vi "Read Active Cell Cell Justification.vi"(8 "error in (no error)":errorcluster, 11 "TreeControl.lvclass in":refnum<class "TreeControl.lvclass">) -> (0 "error out":errorcluster, 2 "CellJustify":enum16{"Left", "Center", "Right"}(ring), 3 "TreeControl.lvclass out":refnum<class "TreeControl.lvclass">)   [LabVIEW 2015, in "TreeControl.lvclass"]
uses:
  TreeControl.lvclass
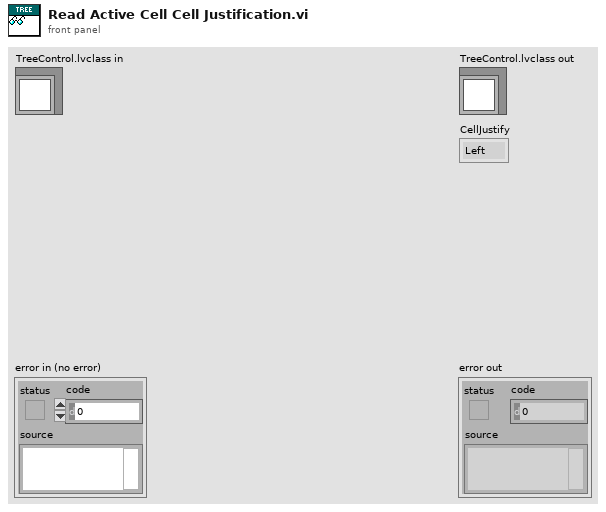
[diagram p1: front panel]
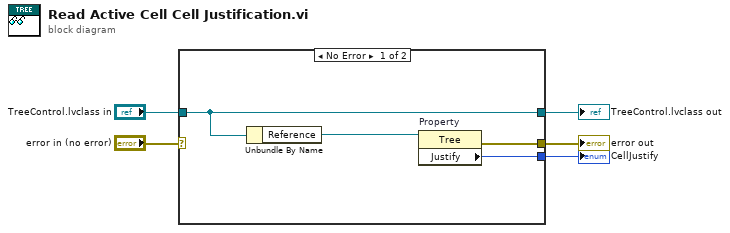
[diagram p0: block diagram]
diagram:
  n1 = case shown="No Error" "error in (no error)" {
    selector: "error in (no error)" -> [_ w11]
    tunnel: [w8 w11] -> w4
    tunnel: [w7 w10] -> w2
    tunnel: "TreeControl.lvclass in" -> [w7 w10]
    tunnel: [w9 _] -> w1
    frame No Error {
      n2 = Unbundle By Name(w7) -> ("Reference"=w6:refnum<vi>)
      n3 = property on="Property" class="Tree"(reference=w6) -> (error out=w8:errorcluster, "Justify"=w9:enum16{"Left", "Center", "Right"})  [unwired: 1 in, 1 out]
    }
    frame Error {
    }
  }
  "error out" <- w4
  "TreeControl.lvclass out" <- w2
  "CellJustify" <- w1
